vi "Stop.vi"(6 "timeout in ms (-1)":i32=-1, 8 "error in (no error)":errorcluster, 10 "Shared Key":string, 11 "SMO":refnum<class "SMO.lvclass">) -> (0 "error out":errorcluster, 3 "SMO out":refnum<class "SMO.lvclass">)   [LabVIEW 2013, in "SMO.lvclass"]
doc: "This method signal all the running processes to shutdown.\n\n<b>ms timeout</b> is the max amount of time allowed for the process to shutdown before an error is reported. <b>ms timeout</b> default is -1 = never times out\n\nNote 01: This method is overridable by descendant\nNote 02: When overridden, Call Parent Method is required\n\n---------------------------------------------------------------\nJKI State Machine Objects™\nhttp://jki.net/state-machine-objects/\nCopyright (C) 2005-2015, JKI <info@jki.net>\nALL RIGHTS RESERVED"
uses:
  SMO.lvclass
panel:
  # "For instructions on how to use the JKI State Machine Objects, examples and video tutorials, visit:\nhttp://jki.net/state-machine-objects/\n\nJKI State Machine Objects™\nhttp://jki.net/state-machine-objects/\nCopyright (C) 2005-2015, JKI <info@jki.net>\nALL RIGHTS RESERVED"
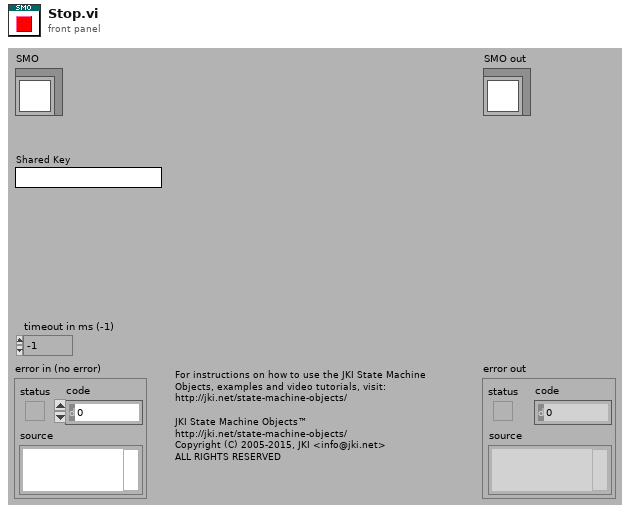
[diagram p1: front panel]
types:
  T1 = typedef "SMO.lvclass/SMOState --Enum.ctl" = enum16{"unknown", "Created", "Started", "Stopped"}
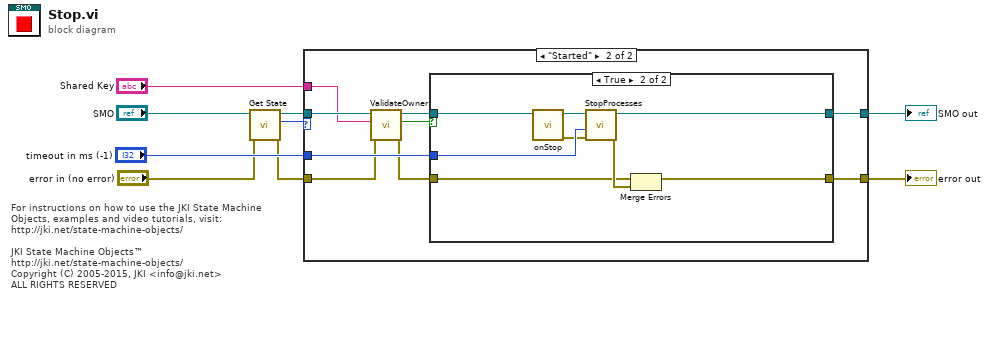
[diagram p0: block diagram]
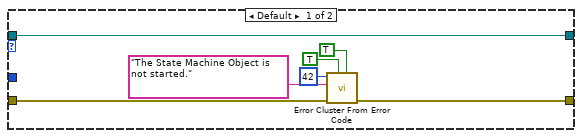
[diagram p2: hidden frame]
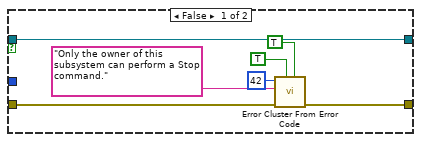
[diagram p3: hidden frame]
diagram:
  # "For instructions on how to use the JKI State Machine Objects, examples and video tutorials, visit:\nhttp://jki.net/state-machine-objects/\n\nJKI State Machine Objects™\nhttp://jki.net/state-machine-objects/\nCopyright (C) 2005-2015, JKI <info@jki.net>\nALL RIGHTS RESERVED"
  n1 = call "Get State.vi"("error in (no error)"="error in (no error)", "SMO"="SMO") -> ("error out"=w3:errorcluster, "SMO State"=w2:T1, "SMO out"=w5:refnum<class "SMO.lvclass">)  [unwired: 7 in]
  n2 = case shown="\"Started\"" w2 {
    tunnel: [w16 w25] -> w9
    tunnel: "timeout in ms (-1)" -> [_ w24]
    tunnel: [w10 w23] -> w7
    tunnel: w5 -> [w16 w22]
    tunnel: w3 -> [w12 w21]
    tunnel: "Shared Key" -> [_ w18]
    frame Default {
      n3 = call <vilib>:"Error Cluster From Error Code.vi"("is warning? (False)"=TRUE, "show call chain? (False)"=TRUE, "error in (no error)"=w12, "error message (\"\")"="The State Machine Object is not started." ("source"), "error code (0)"=42) -> ("error out"=w10:errorcluster)  [unwired: 4 in]
    }
    frame "Started" {
      n4 = call "ValidateOwner.vi"("error in (no error)"=w21, "Shared Key"=w18, "SMO in"=w22) -> ("error out"=w20:errorcluster, "key matched"=w17:bool, "SMO out"=w19:refnum<class "SMO.lvclass">)  [unwired: 6 in]
      n5 = case shown="True" w17 {
        tunnel: [w32 w40] -> w25
        tunnel: w24 -> [_ w39]
        tunnel: [w27 w38] -> w23
        tunnel: w20 -> [w26 w34]
        tunnel: w19 -> [w32 w33]
        frame False {
          n6 = call <vilib>:"Error Cluster From Error Code.vi"("is warning? (False)"=TRUE, "show call chain? (False)"=TRUE, "error in (no error)"=w26, "error message (\"\")"="Only the owner of this subsystem can perform a Stop command." ("source"), "error code (0)"=42) -> ("error out"=w27:errorcluster)  [unwired: 4 in]
        }
        frame True {
          n7 = call-dynamic "onStop.vi"("SMO"=w33) -> ("error out"=w35:errorcluster, "SMO out"=w37:refnum<class "SMO.lvclass">)  [unwired: 9 in]
          n8 = call "StopProcesses.vi"("error in (no error)"=w35, "timeout in ms (-1)"=w39, "SMO"=w37) -> ("error out"=w36:errorcluster, "SMO out"=w40:refnum<class "SMO.lvclass">)  [unwired: 7 in]
          n9 = Merge Errors(w34, w36) -> (w38:errorcluster)
        }
      }
    }
  }
  "error out" <- w7
  "SMO out" <- w9
